vi "sinewavercontrols.vi"() -> ()   [LabVIEW 2014, in "examples.lvlib"]
uses:
  vis/tango_vi.llb/_TangoState_t.ctl
  examples.lvlib
  vis/tango_vi.llb/tango.lvlib
panel:
  out "WaveForm":dbl[](array[numeric])
  in  "DeviceState":T1=enum."UNKNOWN"
  out "WavePoint":dbl
  in  "NoiseAmplitude":dbl=0.6 caption="Noise amplitude"
  in  "Reset Signal":bool
  in  "Phase":dbl
  in  "Offset":dbl
  in  "Amplitude":dbl=1.0
  in  "Frequency":dbl=10.8 format="%#_13g"
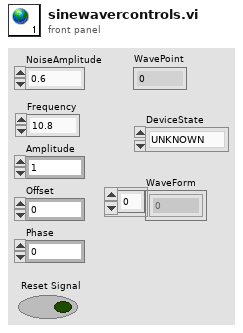
[diagram p1: front panel]
types:
  T1 = typedef "tango.lvlib/_TangoState_t.ctl" = enum32{"ON", "OFF", "CLOSE", "OPEN", "INSERT", "EXTRACT", "MOVING", "STANDBY", "FAULT", "INIT", "RUNNING", "ALARM", "DISABLE", "UNKNOWN"}
diagram:
